vi "FindTopAndBottomEdges (SubVI).vi"(0 "Calibrated Image Array":T1[](array[typedef]), 1 "Fit Options":T8={"Number of Lines"=1, "Type"=enum."Best Edge Rake", "Min. Score"=20.0, "Max. Score"=1000.0, "Orientation"=0.0, "Angle Range"=45.0, "Angle Tolerance"=1.0, "Step Size"=196, "Min. SNR (db)"=0.0, "Min. Points (%)"=25.0, "Hough Iterations"=5} {"Min. Points (%)" min=0.0 max=100.0; "Min. SNR (db)" min=0.0; "Max. Score" min=0.0 max=1024.0; "Min. Score" min=0.0 max=1024.0 step=1.0}, 5 "Options: Top Edge Search":T7={"Search Direction"=2, "Edge Options"={"Edge Polarity"=0, "Kernel Size"=9, "Width"=3, "Minimum Edge Strength"=17.0, "Interpolation Type"=enum."Bilinear Fixed", "Data Processing Method"=enum."Average"}, "Show Search Area"=TRUE, "Show Search Lines"=TRUE, "Show Edges Found"=TRUE, "Show Result"=TRUE, "Search Area Color"=65280, "Search Lines Color"=255, "Edge Locations Color"=16776960, "Result Color"=16711680, "Overlay Group Name"=""} {"Search Direction" items=["Left to Right", "Right to Left", "Top to Bottom", "Bottom to Top"]; "Edge Options"."Edge Polarity" items=["All Edges", "Rising Edges", "Falling Edges"]; "Edge Options"."Minimum Edge Strength" format="%.2f"; "Edge Options"."Width" step=2; "Edge Options"."Kernel Size" step=2}, 9 "Options: Bottom Edge Search":T7={"Search Direction"=3, "Edge Options"={"Edge Polarity"=0, "Kernel Size"=9, "Width"=3, "Minimum Edge Strength"=17.0, "Interpolation Type"=enum."Bilinear Fixed", "Data Processing Method"=enum."Average"}, "Show Search Area"=TRUE, "Show Search Lines"=TRUE, "Show Edges Found"=TRUE, "Show Result"=TRUE, "Search Area Color"=65280, "Search Lines Color"=255, "Edge Locations Color"=16776960, "Result Color"=16711680, "Overlay Group Name"=""} {"Search Direction" items=["Left to Right", "Right to Left", "Top to Bottom", "Bottom to Top"]; "Edge Options"."Edge Polarity" items=["All Edges", "Rising Edges", "Falling Edges"]; "Edge Options"."Minimum Edge Strength" format="%.2f"; "Edge Options"."Width" step=2; "Edge Options"."Kernel Size" step=2}, 11 "error in (no error)":errorcluster, 12 "Templates path":path=path "C:/Users/Sciolla Lab/Desktop/BNLStaveAssembly-Laura/edgeimagebig.png") -> (4 "Analyzed Image Array":T1[](array[typedef]), 6 "Top Edges":T4(array[cluster]), 8 "Bottom Edges":T4(array[cluster]), 10 "Array of Edge Endpoint Arrays":sgl[][][](array[numeric]), 13 "Center Top Coords":dbl[][](array[numeric]), 14 "Center Bottom Coords":dbl[][](array[numeric]), 15 "error in (no error) 2":errorcluster)   [LabVIEW 2016]
uses:
  <vilib>/vision/Measure.llb/Straight Edge Options.ctl
  <vilib>/vision/Measure.llb/Straight Edge Process.ctl
  <vilib>/vision/Measure.llb/Edge Options.ctl
  <vilib>/vision/Measure.llb/Edge Polarity.ctl
  <vilib>/vision/Image Controls.llb/IMAQ Image.ctl
  <vilib>/vision/NI_Vision_Development_Module.lvlib
panel:
  out "Pattern Match Position 2":dbl[](array[numeric])
  out "Pattern Match Position":dbl[](array[numeric])
  out "Template Image 2":T1
  in  "Search Rect":T2={"Left"=0, "Top"=0, "Right"=2147483647, "Bottom"=2147483647, "Rotation"=0.0} {"Rotation" format="%.2f"; "Left" scale=0.0..1024.0; "Right" scale=0.0..1024.0}
  in  "Pattern Match Settings":T3={"Algorithm"=2, "Number of Matches Requested"=1, "Minimum Match Score"=800.0, "SubPixel Accuracy"=TRUE, "Rotation Angle Ranges"=[{"Start"=0.0, "End"=0.0}], "Show Search Area"=FALSE, "Show Result"=TRUE} {"Rotation Angle Ranges"."End" format="%.1f"; "Rotation Angle Ranges"."Start" format="%.1f"; "Minimum Match Score" min=0 max=1000 format="%.2f"; "Number of Matches Requested" min=1; "Algorithm" items=["All", "Low Discrepancy Sampling", "Grayscale Value Pyramid", "Gradients Pyramid"]}
  out "Template Image":T1
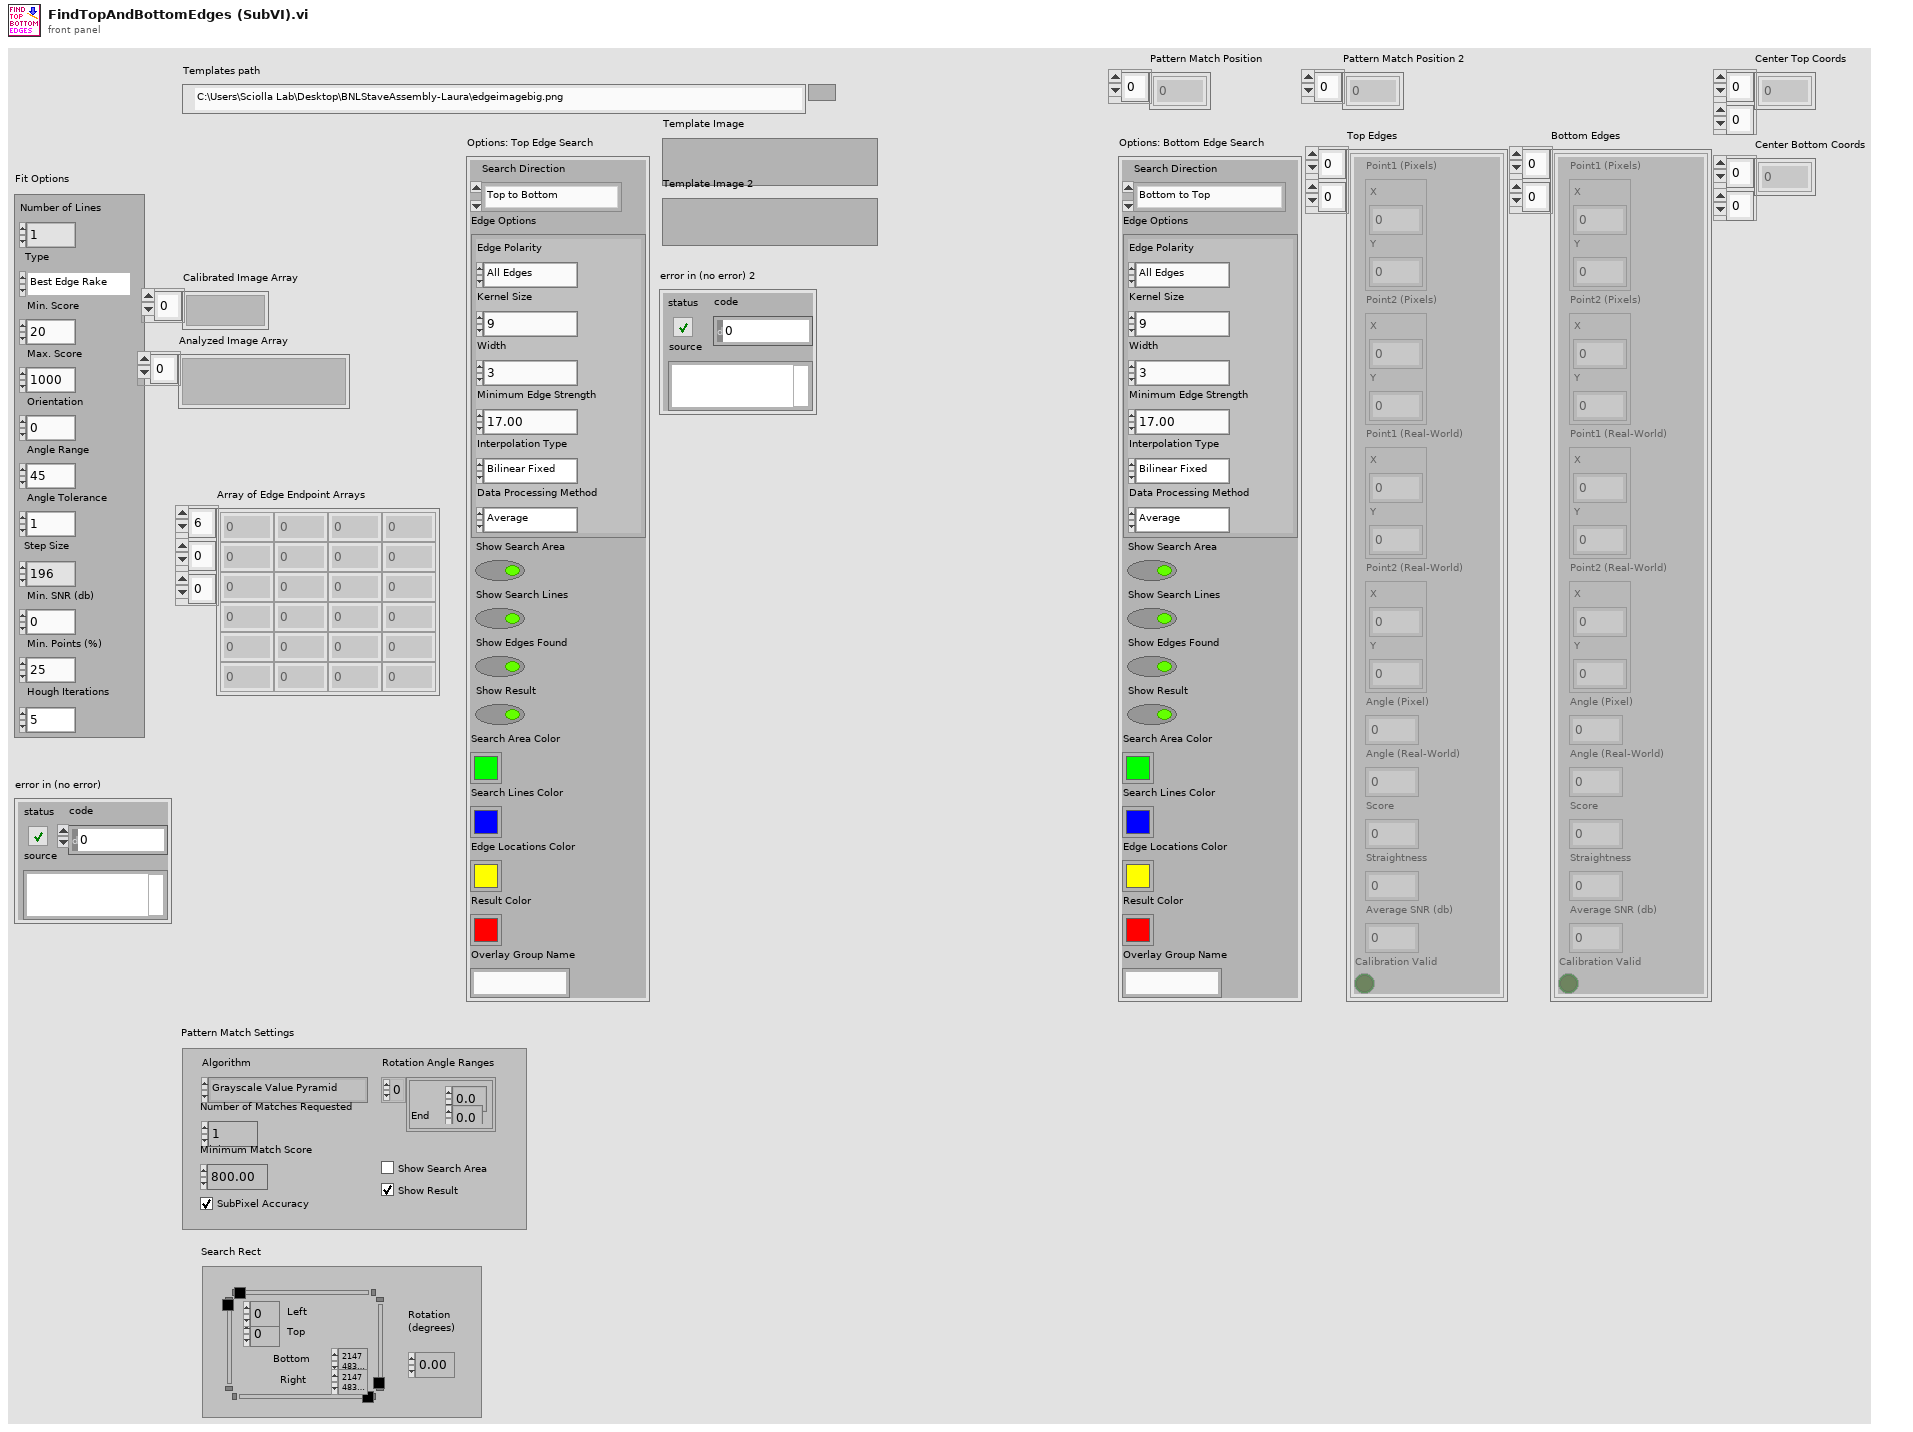
[diagram p1: front panel]
types:
  T1 = typedef "IMAQ Image.ctl" = refnum<image>
  T2 = typedef "IMAQ Rectangle" = cluster{"Left":i32, "Top":i32, "Right":i32, "Bottom":i32, "Rotation":dbl}
  T3 = cluster{"Algorithm":i32, "Number of Matches Requested":i32, "Minimum Match Score":sgl, "SubPixel Accuracy":bool, "Rotation Angle Ranges":cluster{"Start":sgl, "End":sgl}[], "Show Search Area":bool, "Show Result":bool}
  T4 = cluster{"Point1 (Pixels)":cluster{"X":sgl, "Y":sgl}, "Point2 (Pixels)":cluster{"X":sgl, "Y":sgl}, "Point1 (Real-World)":cluster{"X":sgl, "Y":sgl}, "Point2 (Real-World)":cluster{"X":sgl, "Y":sgl}, "Angle (Pixel)":dbl, "Angle (Real-World)":dbl, "Score":dbl, "Straightness":dbl, "Average SNR (db)":dbl, "Calibration Valid":bool}[][]
  T5 = typedef "Edge Options.ctl" = cluster{"Edge Polarity":T6, "Kernel Size":u32, "Width":u32, "Minimum Edge Strength":sgl, "Interpolation Type":enum32{"Zero Order", "Bilinear", "Quadratic", "Cubic", "Bilinear Fixed"}, "Data Processing Method":enum32{"Average", "Median"}}
  T6 = typedef "Edge Polarity.ctl" = u32
  T7 = cluster{"Search Direction":u32, "Edge Options":T5, "Show Search Area":bool, "Show Search Lines":bool, "Show Edges Found":bool, "Show Result":bool, "Search Area Color":u32, "Search Lines Color":u32, "Edge Locations Color":u32, "Result Color":u32, "Overlay Group Name":string}
  T8 = typedef "Straight Edge Options.ctl" = cluster{"Number of Lines":i32, "Type":T9, "Min. Score":dbl, "Max. Score":dbl, "Orientation":dbl, "Angle Range":dbl, "Angle Tolerance":dbl, "Step Size":u32, "Min. SNR (db)":dbl, "Min. Points (%)":dbl, "Hough Iterations":i32}
  T9 = typedef "Straight Edge Process.ctl" = enum32{"First Edge Rake", "Best Edge Rake", "Hough Edge Rake", "First Edge Projection", "Best Edge Projection"}
  T10 = cluster{"Global Rectangle":i32[], cluster{"ID":enum32{"External", "Internal"}, "Type":u32, "Coordinates":i32[]}[]}
  T11 = cluster{"Point1 (Pixels)":cluster{"X":sgl, "Y":sgl}, "Point2 (Pixels)":cluster{"X":sgl, "Y":sgl}, "Point1 (Real-World)":cluster{"X":sgl, "Y":sgl}, "Point2 (Real-World)":cluster{"X":sgl, "Y":sgl}, "Angle (Pixel)":dbl, "Angle (Real-World)":dbl, "Score":dbl, "Straightness":dbl, "Average SNR (db)":dbl, "Calibration Valid":bool}[]
  T12 = cluster{"Point1 (Pixels)":cluster{"X":sgl, "Y":sgl}, "Point2 (Pixels)":cluster{"X":sgl, "Y":sgl}, "Point1 (Real-World)":cluster{"X":sgl, "Y":sgl}, "Point2 (Real-World)":cluster{"X":sgl, "Y":sgl}, "Angle (Pixel)":dbl, "Angle (Real-World)":dbl, "Score":dbl, "Straightness":dbl, "Average SNR (db)":dbl, "Calibration Valid":bool}
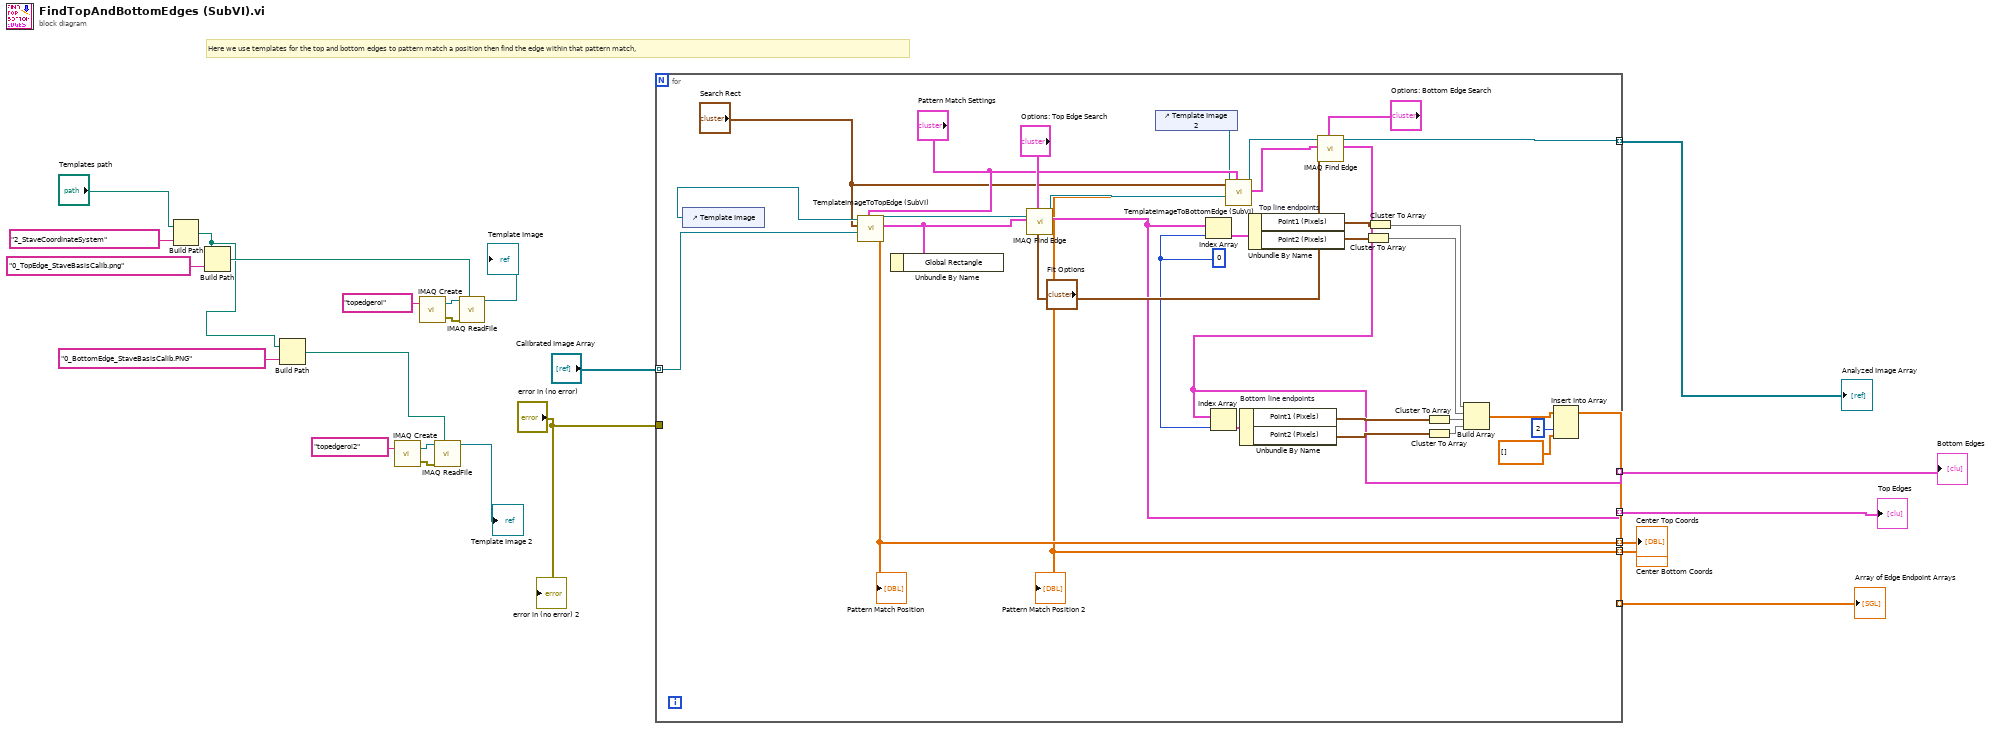
[diagram p0: block diagram]
diagram:
  # "Here we use templates for the top and bottom edges to pattern match a position then find the edge within that pattern match,"
  n1 = Build Path(base path="Templates path", name or relative path="2_StaveCoordinateSystem") -> (appended path=w3:path)
  n2 = Build Path(base path=w3, name or relative path="0_TopEdge_StaveBasisCalib.png") -> (appended path=w4:path)
  n3 = Build Path(base path=w3, name or relative path="0_BottomEdge_StaveBasisCalib.PNG") -> (appended path=w6:path)
  n4 = call "IMAQ Create"("Image Name"="topedgeroi2") -> ("New Image"=w12:T1, "error out"=w13:errorcluster)  [unwired: 4 in]
  n5 = call "IMAQ Create"("Image Name"="topedgeroi") -> ("New Image"=w16:T1, "error out"=w17:errorcluster)  [unwired: 4 in]
  n6 = call "IMAQ ReadFile"("File Path"=w6, "error in (no error)"=w13, "Image"=w12) -> ("Image Out"=→"Template Image 2":T1)  [unwired: 4 in, 4 out]
  n7 = call "IMAQ ReadFile"("File Path"=w4, "error in (no error)"=w17, "Image"=w16) -> ("Image Out"=→"Template Image":T1)  [unwired: 4 in, 4 out]
  n8 = for {
    tunnel: "Calibrated Image Array" -> [w34] mode=indexing
    tunnel: "error in (no error)" -> [_]
    tunnel: [w53] -> w23 mode=indexing
    tunnel: [w35] -> w21 mode=indexing
    tunnel: [w38] -> w20 mode=indexing
    tunnel: [w37] -> w19 mode=indexing
    tunnel: [w25] -> w2 mode=indexing
    tunnel: [w24] -> w1 mode=indexing
    w52 = 0 ("index")
    n9 = control-ref of="Template Image"() -> (w28:refnum<vi>)
    n10 = call "TemplateImageToTopEdge (SubVI).vi"("Pattern Match Settings"="Pattern Match Settings", "Calibrated Image"=w34, "Search Rect"="Search Rect", "GenClassTagFlatRef in"=w28) -> ("Pattern Match Position"=w25:dbl[], "ROI Descriptor after matches"=w26:T10, "Refnum out"=w36:T1)  [unwired: 4 in, 1 out]
    "Pattern Match Position" <- w25
    n11 = Unbundle By Name(w26) -> ()  [unwired: 1 out]
    n12 = call "IMAQ Find Edge"("Line Fit Options"="Fit Options", "Options"="Options: Top Edge Search", "ROI Descriptor"=w26, "Image"=w36) -> ("Straight Edges"=w35:T11, "Image Out"=w33:T1)  [unwired: 4 in, 2 out]
    n13 = control-ref of="Template Image 2"() -> (w30:refnum<vi>)
    n14 = Index Array(array=w35, index=w52) -> (element=w51:T12)
    n15 = call "TemplateImageToBottomEdge (SubVI).vi"("Pattern Match Settings"="Pattern Match Settings", "Calibrated Image"=w33, "Search Rect"="Search Rect", "GenClassTagFlatRef in"=w30) -> ("Pattern Match Position"=w24:dbl[], "ROI Descriptor after matches"=w29:T10, "Refnum out"=w32:T1)  [unwired: 4 in, 1 out]
    "Pattern Match Position 2" <- w24
    n16 = Unbundle By Name "Top line endpoints"(w51) -> ("Point1 (Pixels)"=w49:cluster{"X":sgl, "Y":sgl}, "Point2 (Pixels)"=w48:cluster{"X":sgl, "Y":sgl})
    n17 = call "IMAQ Find Edge"("Line Fit Options"="Fit Options", "Options"="Options: Bottom Edge Search", "ROI Descriptor"=w29, "Image"=w32) -> ("Straight Edges"=w38:T11, "Image Out"=w53:T1)  [unwired: 4 in, 2 out]
    n18 = Index Array(array=w38, index=w52) -> (element=w50:T12)
    n19 = Unbundle By Name "Bottom line endpoints"(w50) -> ("Point1 (Pixels)"=w41:cluster{"X":sgl, "Y":sgl}, "Point2 (Pixels)"=w42:cluster{"X":sgl, "Y":sgl})
    n20 = Cluster To Array(cluster=w48) -> (array=w46:sgl[])
    n21 = Cluster To Array(cluster=w49) -> (array=w47:sgl[])
    n22 = Cluster To Array(cluster=w41) -> (array=w40:sgl[])
    n23 = Cluster To Array(cluster=w42) -> (array=w39:sgl[])
    n24 = Build Array(w47, w46, w40, w39) -> (w45:sgl[][])
    n25 = Insert Into Array(array=w45, index (col)=2 ("disabled index (col)"), new element=sgl[] [] ("new element/subarray")) -> (w37:sgl[][])  [unwired: 1 in]
  }
  "Analyzed Image Array" <- w23
  "Top Edges" <- w21
  "Bottom Edges" <- w20
  "Array of Edge Endpoint Arrays" <- w19
  "Center Top Coords" <- w2
  "Center Bottom Coords" <- w1
  "error in (no error) 2" <- "error in (no error)"
